vi "Global_morevar.vi"() -> ()   [LabVIEW 2014]
panel:
  out "dir cmd out":dbl
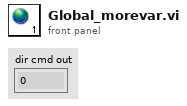
[diagram p1: front panel]
diagram:
